vi "ma_Limit Test Outside.vi"(5 "x0":dbl format="%0.2f", 7 "dx":dbl=1.0 format="%0.2f", 8 "limit test config":T2={"pass region"=0, "include UL"=TRUE, "include LL"=TRUE} {"pass region" items=["inside limits", "outside limits"]}, 9 "lower":dbl[](array[numeric]) format="%0.2f", 10 "upper":dbl[](array[numeric]) format="%0.2f", 11 "signal":dbl[](array[numeric]) format="%0.2f") -> (0 "clearance":T1 {"min clearance" format="%.2f"; "clearance LL" format="%.2f"; "clearance UL" format="%.2f"}, 1 "failures":cluster{"x values":dbl[], "y values":dbl[]} {"y values" format="%.2f"; "x values" format="%.2f"}, 2 "test results":bool[](array[boolean]), 3 "Y":dbl[](array[numeric]) format="%0.2f")   [LabVIEW 2020, in "NI_MAPro.lvlib"]
uses:
  NI_MAPro.lvlib
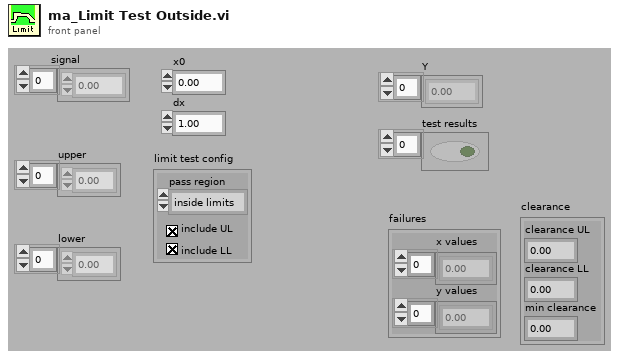
[diagram p1: front panel]
types:
  T1 = cluster{"clearance UL":dbl, "clearance LL":dbl, "min clearance":dbl}
  T2 = cluster{"pass region":i32, "include UL":bool, "include LL":bool}
  T3 = cluster{"clearanceUL":dbl, "clearanceUL":dbl, dbl}
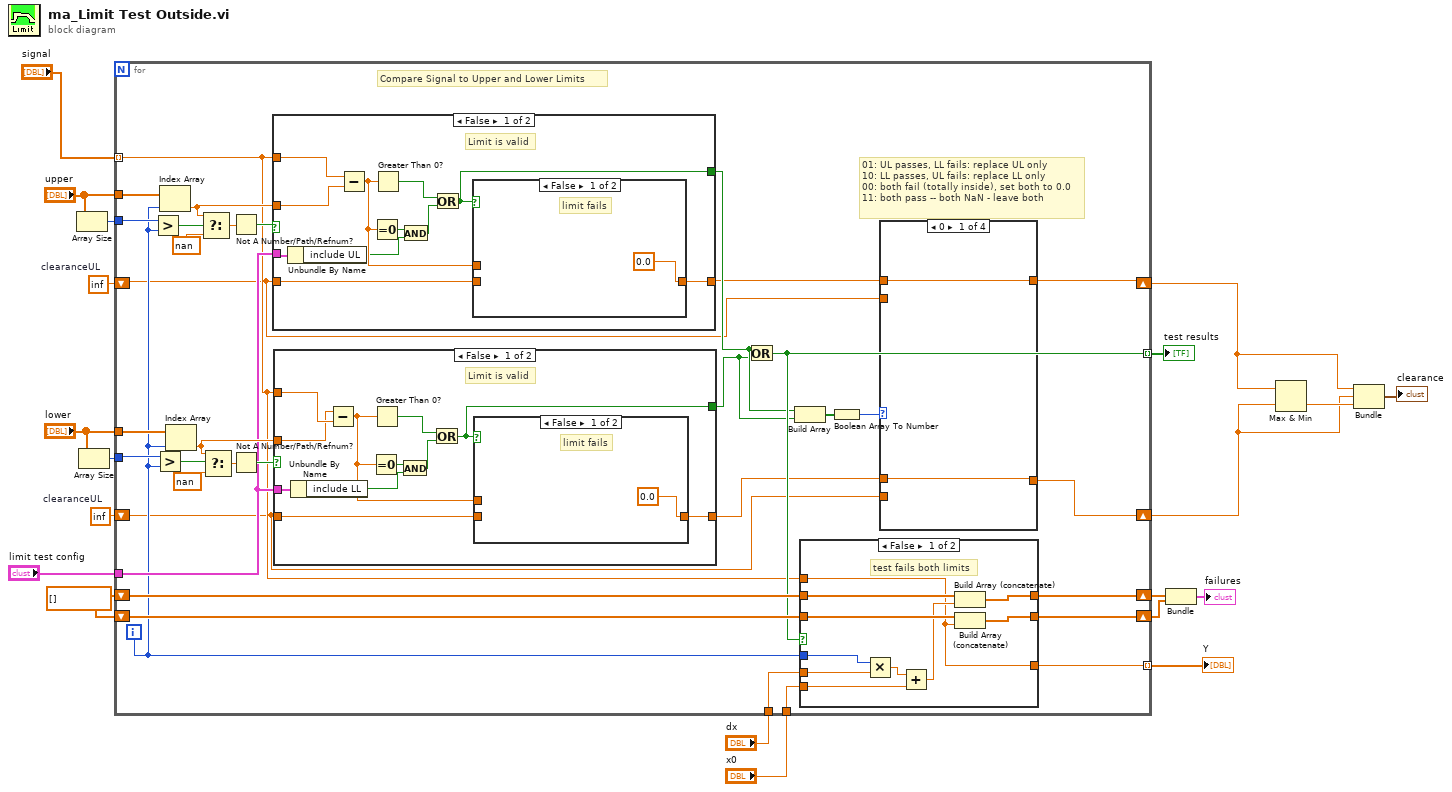
[diagram p0: block diagram]
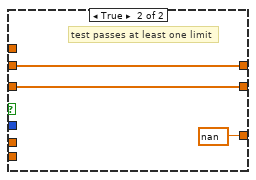
[diagram p5: hidden frame]
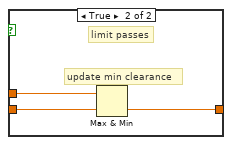
[diagram p6: hidden frame]
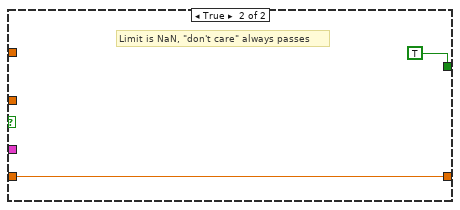
[diagram p7: hidden frame]
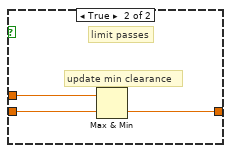
[diagram p8: hidden frame]
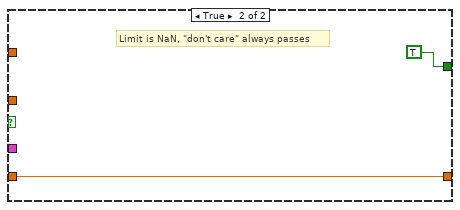
[diagram p9: hidden frame]
diagram:
  w13 = dbl[] [] ("x values")
  w14 = inf  # clearanceUL
  w16 = inf  # clearanceUL
  n1 = Array Size(array="upper") -> (size(s)=w18:i32)
  n2 = Array Size(array="lower") -> (size(s)=w17:i32)
  n3 = for {
    tunnel: "upper" -> [w49]
    tunnel: "signal" -> [w33] mode=indexing
    tunnel: "lower" -> [w48]
    tunnel: w18 -> [w55]
    tunnel: w17 -> [w51]
    tunnel: "limit test config" -> [w41]
    shift-right: [w26] -> w7
    shift-left: w16 -> [w25]
    shift-right: [w23] -> w6
    shift-left: w14 -> [w24]
    shift-right: [w37] -> w12
    shift-left: w13 -> [w40]
    shift-right: [w36] -> w11
    shift-left: w13 -> [w39]
    tunnel: [w35] -> w9 mode=indexing
    tunnel: [w34] -> w4 mode=indexing
    tunnel: "dx" -> [w22]
    tunnel: "x0" -> [w21]
    i -> [w38]
    # "01: UL passes, LL fails: replace UL only\n10: LL passes, UL fails: replace LL only\n00: both fail (totally inside), set both to 0.0\n11: both pass -- both NaN - leave both"
    # "Compare Signal to Upper and Lower Limits"
    n4 = Greater?(x=w55, y=w38) -> (0:w54:bool)
    n5 = Greater?(x=w51, y=w38) -> (0:w50:bool)
    n6 = Index Array(array=w49, index=w38) -> (element=w45:dbl)
    n7 = Index Array(array=w48, index=w38) -> (element=w42:dbl)
    n8 = Select(t=w45, s=w54, f=nan ("t")) -> (s? t:f=w47:dbl)
    n9 = Select(t=w42, s=w50, f=nan ("t")) -> (s? t:f=w44:dbl)
    n10 = Not A Number/Path/Refnum?(number/path/refnum=w47) -> (NaN/Path/Refnum?=w46:bool)
    n11 = Not A Number/Path/Refnum?(number/path/refnum=w44) -> (NaN/Path/Refnum?=w43:bool)
    n12 = case shown="False" w46 {
      tunnel: w45 -> [w104 _]
      tunnel: w33 -> [w103 _]
      tunnel: w41 -> [w95 _]
      tunnel: w25 -> [w99 w110]
      tunnel: [w97 w110] -> w28
      tunnel: [w94 TRUE] -> w31
      frame False {
        # "Limit is valid"
        n13 = Unbundle By Name(w95) -> ("include UL"=w96:bool)
        n14 = Subtract(x=w103, y=w104) -> (x-y=w98:dbl)
        n15 = Equal To 0?(x=w98) -> (x = 0?=w102:bool)
        n16 = Greater Than 0?(x=w98) -> (x > 0?=w101:bool)
        n17 = And(x=w102, y=w96) -> (x .and. y?=w100:bool)
        n18 = Or(x=w101, y=w100) -> (x .or. y?=w94:bool)
        n19 = case shown="False" w94 {
          tunnel: w99 -> [_ w107]
          tunnel: [0.0 w106] -> w97
          tunnel: w98 -> [_ w108]
          frame False {
            # "limit fails"
          }
          frame True {
            # "update min clearance"
            # "limit passes"
            n20 = Max & Min(x=w108, y=w107) -> (min(x,y)=w106:dbl)  [unwired: 1 out]
          }
        }
      }
      frame True {
        # "Limit is NaN, \"don't care\" always passes"
      }
    }
    n21 = case shown="False" w43 {
      tunnel: w42 -> [w77 _]
      tunnel: w33 -> [w87 _]
      tunnel: w24 -> [w83 w93]
      tunnel: [w81 w93] -> w27
      tunnel: w41 -> [w80 _]
      tunnel: [w78 TRUE] -> w30
      frame False {
        # "Limit is valid"
        n22 = Unbundle By Name(w80) -> ("include LL"=w79:bool)
        n23 = Subtract(x=w77, y=w87) -> (x-y=w82:dbl)
        n24 = Equal To 0?(x=w82) -> (x = 0?=w86:bool)
        n25 = Greater Than 0?(x=w82) -> (x > 0?=w85:bool)
        n26 = And(x=w86, y=w79) -> (x .and. y?=w84:bool)
        n27 = Or(x=w85, y=w84) -> (x .or. y?=w78:bool)
        n28 = case shown="False" w78 {
          tunnel: w83 -> [_ w90]
          tunnel: [0.0 w89] -> w81
          tunnel: w82 -> [_ w91]
          frame False {
            # "limit fails"
          }
          frame True {
            # "update min clearance"
            # "limit passes"
            n29 = Max & Min(x=w91, y=w90) -> (min(x,y)=w89:dbl)  [unwired: 1 out]
          }
        }
      }
      frame True {
        # "Limit is NaN, \"don't care\" always passes"
      }
    }
    n30 = Or(x=w31, y=w30) -> (x .or. y?=w35:bool)
    n31 = Build Array(w31, w30) -> (w32:bool[])
    n32 = case shown="False" w35 {
      tunnel: w40 -> [w73 w76]
      tunnel: w39 -> [w72 w75]
      tunnel: w38 -> [w70 _]
      tunnel: w33 -> [w66 _]
      tunnel: [w68 w76] -> w37
      tunnel: [w67 w75] -> w36
      tunnel: [w66 nan] -> w34
      tunnel: w22 -> [w65 _]
      tunnel: w21 -> [w64 _]
      frame False {
        # "test fails both limits"
        n33 = Multiply(x=w70, y=w65) -> (x*y=w71:dbl)
        n34 = Add(x=w71, y=w64) -> (x+y=w69:dbl)
        n35 = Build Array (concatenate)(w73, w69) -> (w68:dbl[])
        n36 = Build Array (concatenate)(w72, w66) -> (w67:dbl[])
      }
      frame True {
        # "test passes at least one limit"
      }
    }
    n37 = Boolean Array To Number(Boolean array=w32) -> (number=w29:u32)
    n38 = case shown="0" w29 {
      tunnel: w28 -> [w57 w59 _ _]
      tunnel: w27 -> [w56 _ w60 _]
      tunnel: [w57 w59 w61 w62] -> w26
      tunnel: w25 -> [_ _ w61 w62]
      tunnel: w24 -> [_ w58 _ w63]
      tunnel: [w56 w58 w60 w63] -> w23
      frame 0 {
      }
      frame 1 {
      }
      frame 2 {
      }
      frame 3, Default {
      }
    }
  }
  "test results" <- w9
  "Y" <- w4
  n39 = Bundle("x values"=w12, "x values"=w11) -> (→"failures":cluster{"x values":dbl[], "x values":dbl[]})  [unwired: 1 out]
  n40 = Max & Min(x=w7, y=w6) -> (min(x,y)=w8:dbl)  [unwired: 1 out]
  n41 = Bundle("clearanceUL"=w7, "clearanceUL"=w6, w8) -> (→"clearance":T3)  [unwired: 1 out]
